vi "XNET.Create.DatabasePath.vi"(8 "error in (no error)":errorcluster, 11 "DB Alias":string) -> (0 "error out":errorcluster, 3 "DB Path":path)   [LabVIEW 2019, in "Diagnostics Addon Shared.lvlib"]
uses:
  Diagnostics Addon Shared.lvlib
  NationalInstruments.VeriStand.Internal
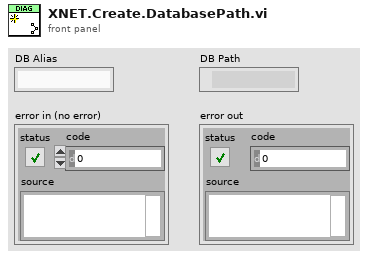
[diagram p1: front panel]
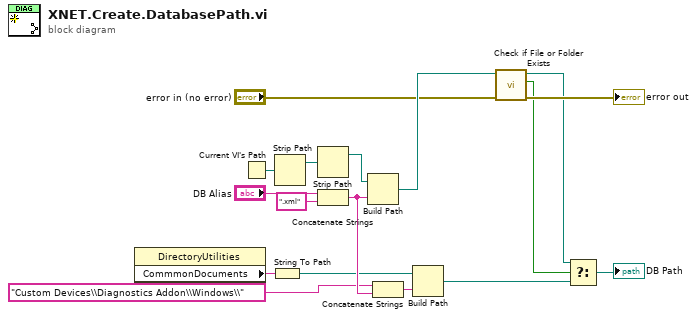
[diagram p0: block diagram]
diagram:
  n1 = property class="DirectoryUtilities"() -> ("CommmonDocuments"=w6:string)  [unwired: 2 in, 2 out]
  n2 = Current VI's Path() -> (path=w3:path)
  n3 = String To Path(string=w6) -> (path=w7:path)
  n4 = Strip Path(path=w3) -> (stripped path=w1:path)  [unwired: 1 out]
  n5 = Strip Path(path=w1) -> (stripped path=w4:path)  [unwired: 1 out]
  n6 = Concatenate Strings("DB Alias", ".xml" ("string")) -> (w10:string)
  n7 = Build Path(base path=w4, name or relative path=w10) -> (appended path=w16:path)
  n8 = Concatenate Strings("Custom Devices\\Diagnostics Addon\\Windows\\" ("name or relative path"), w10) -> (w9:string)
  n9 = Build Path(base path=w7, name or relative path=w9) -> (appended path=w13:path)
  n10 = call <vilib>:"Check if File or Folder Exists.vi"("error in (no error)"="error in (no error)", "path"=w16) -> ("error out"=→"error out":errorcluster, "file or folder exists?"=w11:bool, "dup path"=w12:path)  [unwired: 7 in]
  n11 = Select(t=w12, s=w11, f=w13) -> (s? t:f=→"DB Path":path)
